vi "writer2.vi"() -> ()   [LabVIEW 2010]
uses:
  <vilib>/measure/NI_MABase.lvlib
panel:
  in  "Boolean":bool
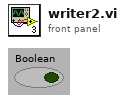
[diagram p1: front panel]
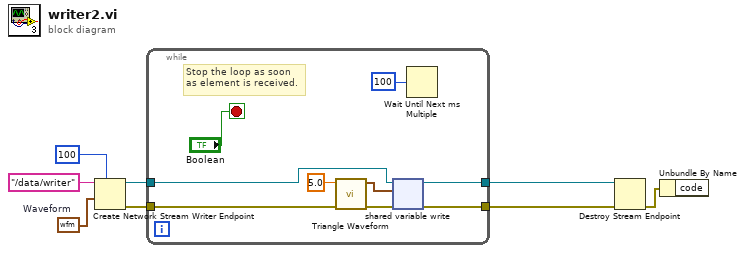
[diagram p0: block diagram]
diagram:
  w5 = waveform(dbl) {"t0"=timestamp(0 s since 1904-01-01), "dt"=1.0, "Y"=[]}  # Waveform
  n1 = Create Network Stream Writer Endpoint(7:100 ("writer buffer size"), 9:w5, 11:"/data/writer" ("writer name")) -> (0:w6:errorcluster, 3:w7:refnum<k21>)  [unwired: 3 in]
  n2 = while {
    tunnel: w7 -> [w17]
    tunnel: w6 -> [w16]
    tunnel: [w15] -> w4
    tunnel: [w14] -> w3
    stop <- "Boolean" stop-if-true
    # "Stop the loop as soon \nas element is received."
    n3 = call <vilib>:"Triangle Waveform.vi"("error in (no error)"=w16, "frequency"=5.0) -> ("error out"=w12:errorcluster, "signal out"=w11:waveform(dbl))  [unwired: 8 in]
    n4 = shared-variable-write(w17, w12, w11) -> (w14:refnum<k21>, w15:errorcluster)  [unwired: 1 in, 1 out]
    n5 = Wait Until Next ms Multiple(millisecond multiple=u32 100 ("milliseconds to wait")) -> ()  [unwired: 1 out]
  }
  n6 = Destroy Stream Endpoint(8:w4, 11:w3) -> (0:w1:errorcluster)
  n7 = Unbundle By Name(w1) -> ()  [unwired: 1 out]
